vi "Main.vi"() -> ()   [LabVIEW 2020]
uses:
  States.ctl
  <vilib>/Instr/_visa.llb/VISA Configure Serial Port (Serial Instr).vi
  <vilib>/Utility/file.llb/Read Delimited Spreadsheet (I64).vi
panel:
  out "Next Control State":T1
  out "Next Com State":enum16{"Initialize", "Send", "Receive", "Error"}(ring)=enum."Receive"
  out "Next Cmd":enum16{"getParm", "inc", "mph", "err"}(ring)
  out "Send Buffer":string
  out "Control Error":errorcluster
  out "Com Error":errorcluster
  out "Missed Msg":u16
  out "Time Left":u32
  out "Inc Changed":bool
  out "Next MPH":u16
  out "Next Duration":u16
  out "Next Inc":u16
  out "PD READ":u8
  out "INC READ":u8
  out "MPH READ":u8
  out "dwell":u16[](array[numeric])
  out "incline":u16[](array[numeric])
  out "time":u16[](array[numeric])
  out "speed":u16[](array[numeric])
  out "input lines":i32
  in  "TestScript":path=path "C:/LabView Computer Backup SEAL2788/DonP_TRM500/FootTimeInc.txt"
  out "read buffer":string
  out "Speed Changed":bool
  in  "Manual Stop":bool
  in  "Serial Port":refnum<visa-resource-name>="COM8"
  out "FootPath":path
  out "FootPathRef":refnum<file>
  out "stopping":bool
  out "Target MPH":u16 max=12 step=1
  out "step":i32
  out "Target INC":u16 max=12 step=1
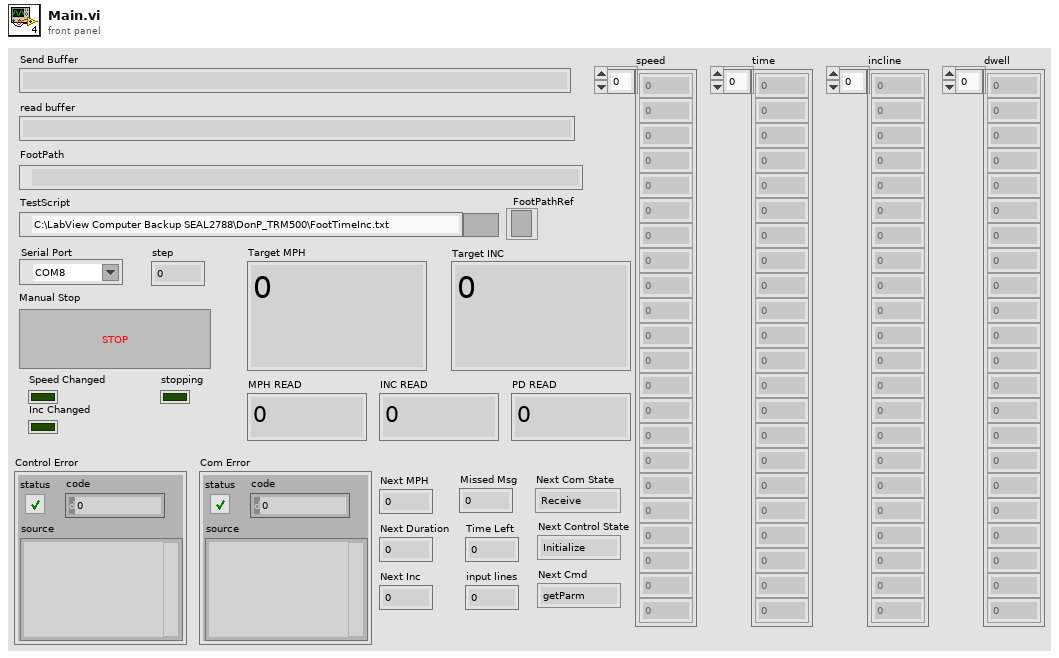
[diagram p1: front panel]
types:
  T1 = typedef "States.ctl" = enum16{"Initialize", "SetTargets", "WaitforMPH", "Dwell", "CheckTiming"}
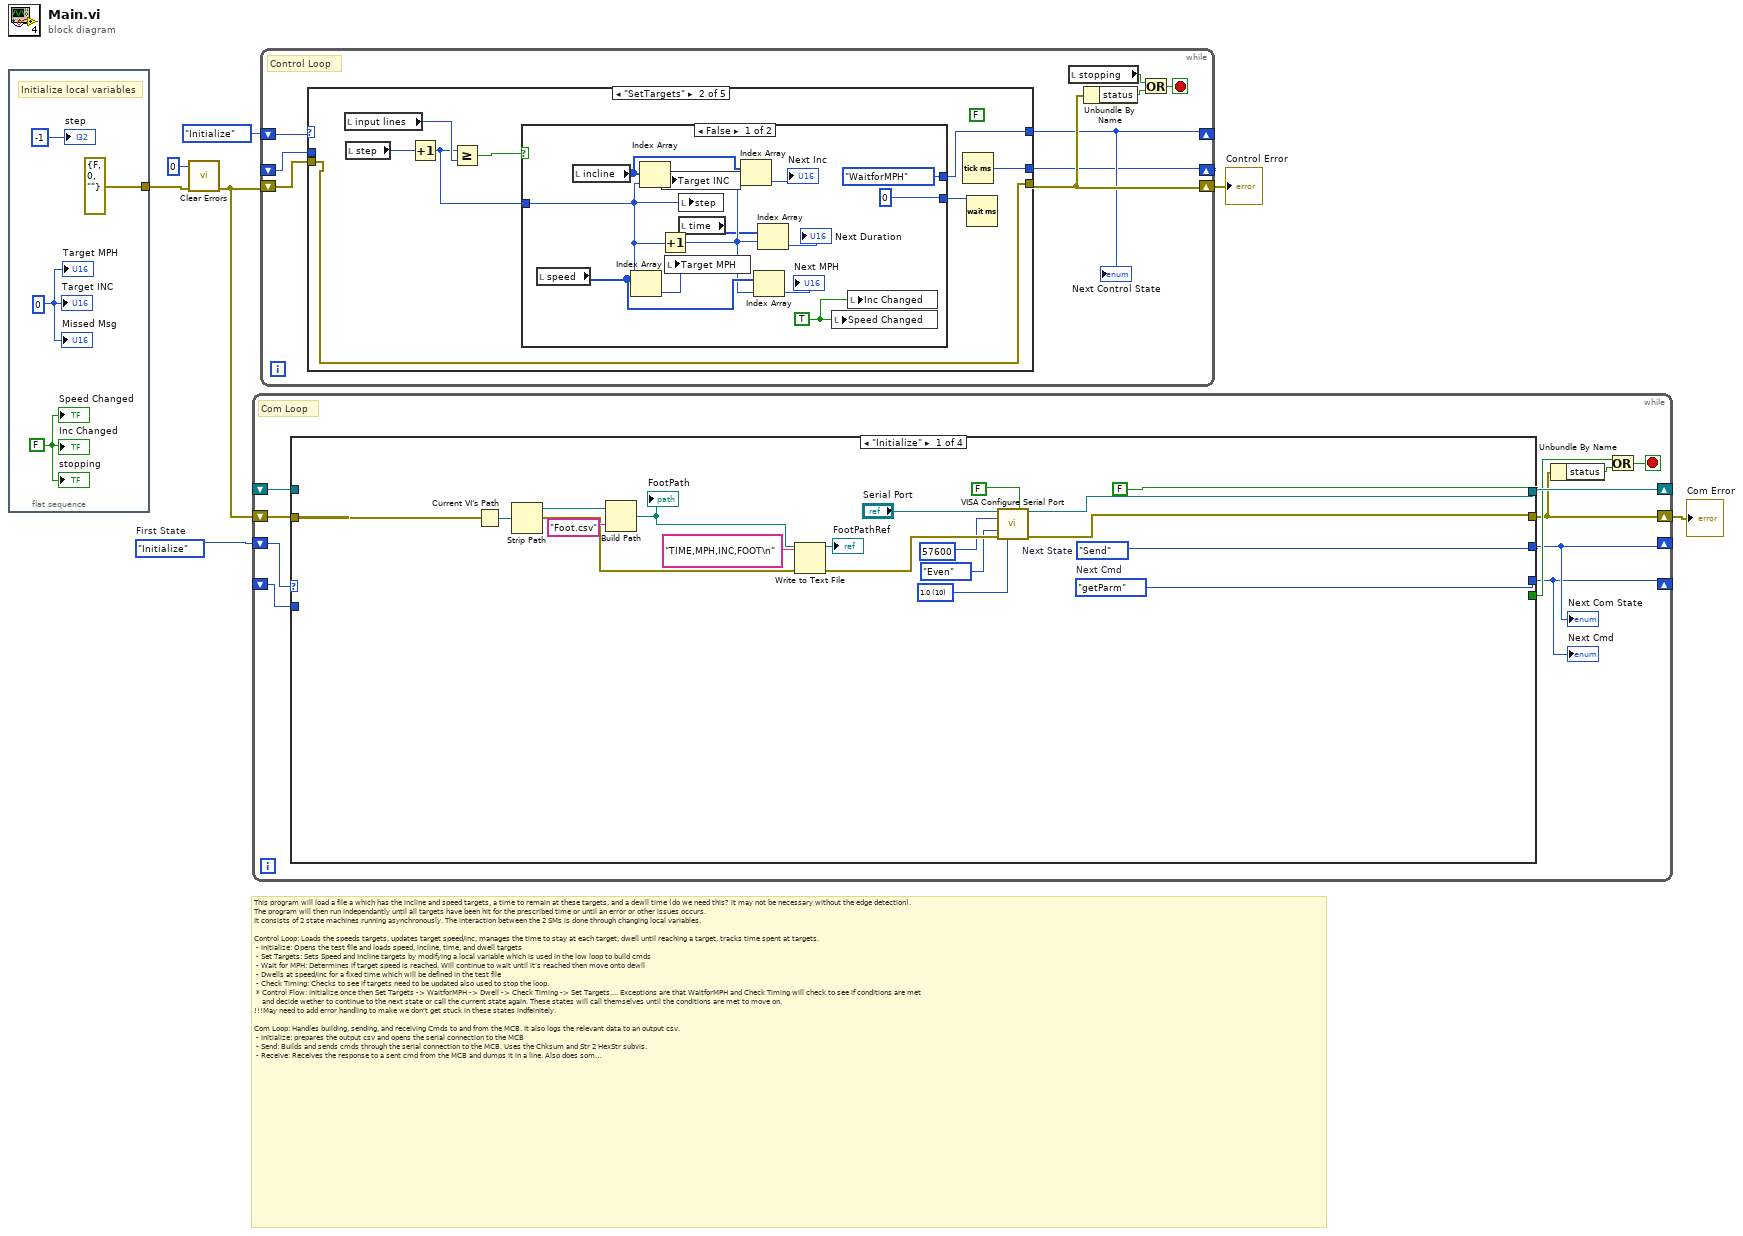
[diagram p0: block diagram]
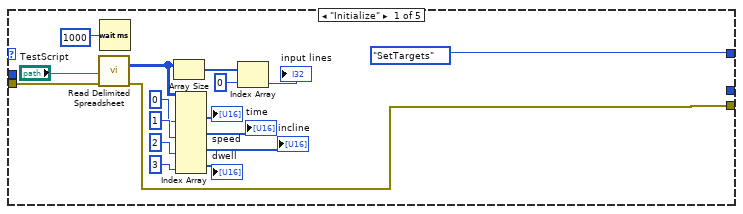
[diagram p2: hidden frame]
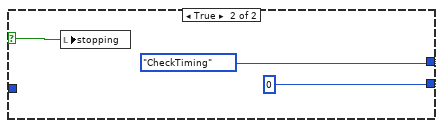
[diagram p3: hidden frame]
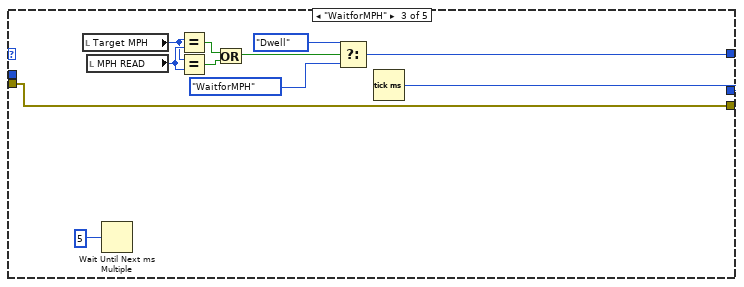
[diagram p4: hidden frame]
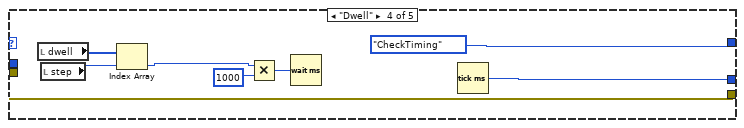
[diagram p5: hidden frame]
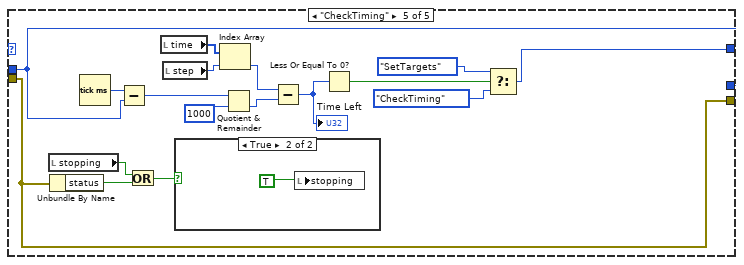
[diagram p6: hidden frame]
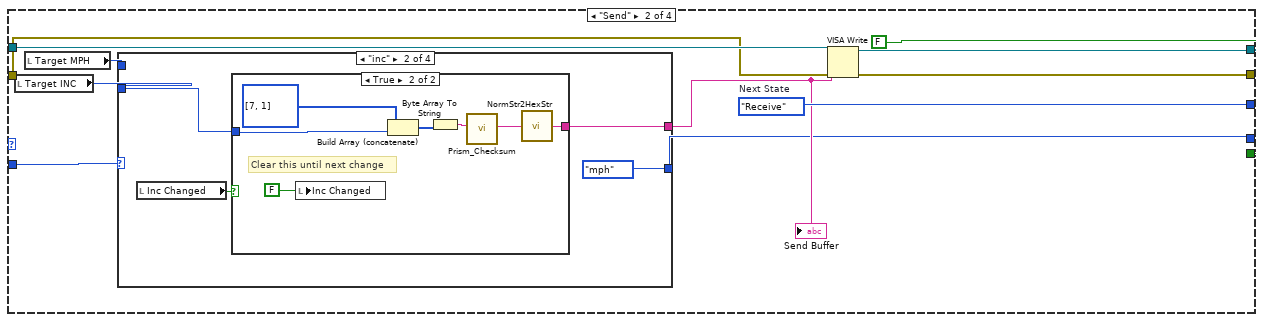
[diagram p8: hidden frame]
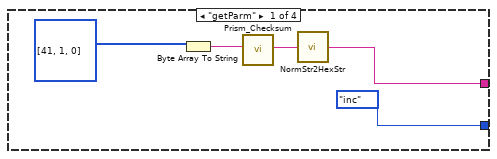
[diagram p9: hidden frame]
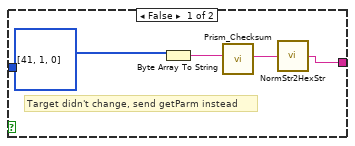
[diagram p10: hidden frame]
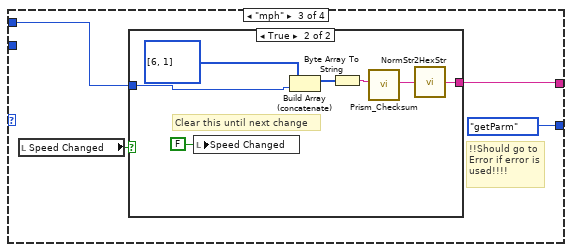
[diagram p11: hidden frame]
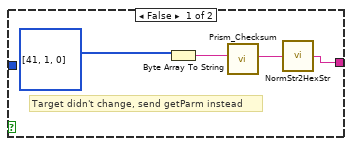
[diagram p12: hidden frame]
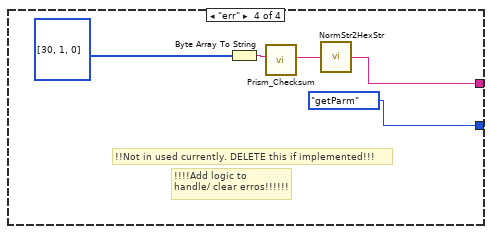
[diagram p13: hidden frame]
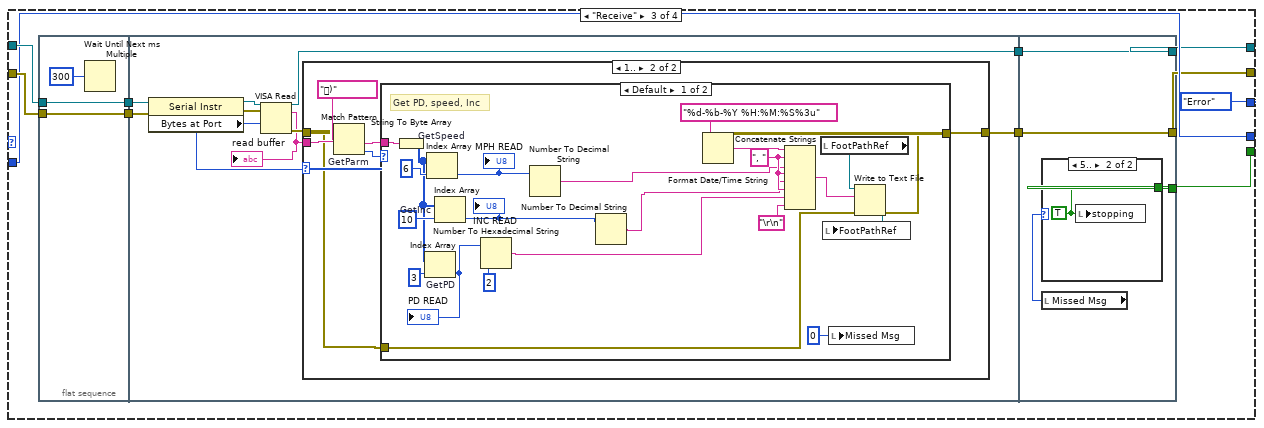
[diagram p14: hidden frame]
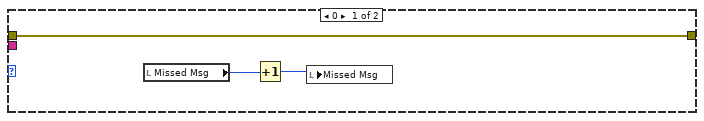
[diagram p15: hidden frame]
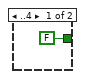
[diagram p17: hidden frame]
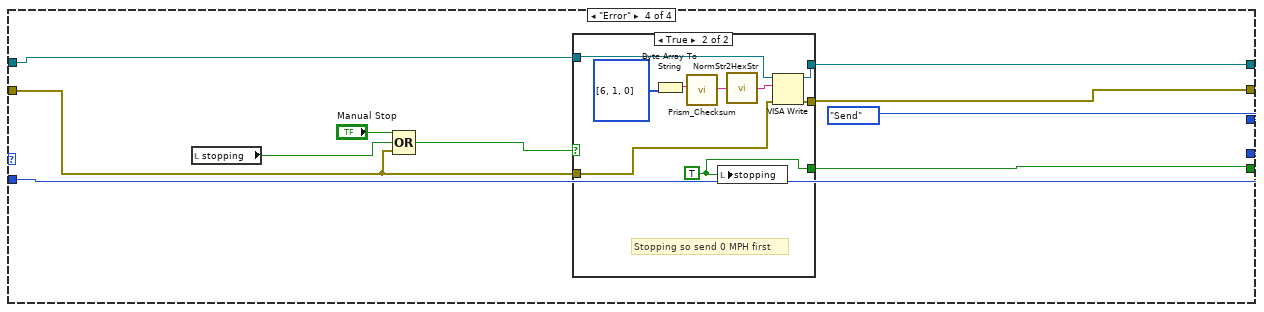
[diagram p18: hidden frame]
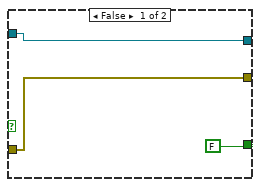
[diagram p19: hidden frame]
diagram:
  w7 = enum16{"Initialize", "Send", "Receive", "Error"}."Initialize"  # First State
  # "This program will load a file a which has the incline and speed targets, a time to remain at these targets, and a dewll time (do we need this? it may not be necessary without the edge detection).\nThe program will then run independantly until all targets have been hit for the prescribed time or until an error or other issues occurs.\nIt consists of 2 state machines running asynchronously. The interaction between the 2 SMs is done through changing local variables.\n\nControl Loop: Loads the speeds targets, updates target speed/inc, manages the time to stay at each target, dwell until reaching a target, tracks time spent at targets. \n - Initialize: Opens the test file and loads speed, incline, time, and dwell targets \n - Set Targets: Sets Speed and Incline targets by modifying a local variable which is used in the low loop to build cmds \n - Wait for MPH: Determines if target speed is reached. Will continue to wait until it's reached then move onto dewll\n - Dwells at speed/inc for a fixed time which will be defined in the test file\n - Check Timing: Checks to see if targets need to be updated also used to stop the loop.\n * Control Flow: Initialize once then Set Targets -> WaitforMPH -> Dwell -> Check Timing -> Set Targets.... Exceptions are that WaitforMPH and Check Timing will check to see if conditions are met\n    and decide wether to continue to the next state or call the current state again. These states will call themselves until the conditions are met to move on. \n!!!May need to add error handling to make we don't get stuck in these states indfeinitely.\n\nCom Loop: Handles building, sending, and receiving Cmds to and from the MCB. It also logs the relevant data to an output csv.\n - Initialize: prepares the output csv and opens the serial connection to the MCB\n - Send: Builds and sends cmds through the serial connection to the MCB. Uses the Chksum and Str 2 HexStr subvis. \n - Receive: Receives the response to a sent cmd from the MCB and dumps it in a line. Also does some analysis of the response to determine current  Speed/inc/person detect\n - Error:  Stops the program. This handles labview errors and will stop the program when one is encounted. It also handles stopping when reaching the end of a test \n * Com Flow: nitialize once then Send -> Receive -> Error -> Send...\n * Send flow: GetParm -> Inc -> MPH -> GetParm etc. Exception is that it will check first to see if the target changed and if it hasn't will send getParm Instead\n!!!May need to add error handling in which case the flow should be GetParm -> MPH -> Inc -> Err -> GetParm....\n\nFiles:\n1 input file which contains the test script to run. Format: Speed, Time, Inc, Dwell. Time = time to stay at target speed/inc. Dwell = a fixed time to wait after reaching targets and before starting the Time counter. This is used to make sure the speed stablizes before starting the Time counter.\n1 output file which contains Timestamp, Speed, Incline, and a flag for if person is detected (0 = No, 1 = Yes). Format: TIME,MPH,INC,FOOT"
  n1 = flat-sequence {
    tunnel: [errorcluster {"status"=FALSE, "code"=0, "source"=""} ("error constant")] -> w3
    frame #0 {
      w9 = FALSE ("Inc Changed")
      w8 = u16 0 ("MPH")
      # "Initialize local variables"
      "stopping" <- w9
      "Target MPH" <- w8
      "step" <- -1 ("step")
      "Target INC" <- w8
      "Speed Changed" <- w9
      "Inc Changed" <- w9
      "Missed Msg" <- w8
    }
  }
  n2 = call <vilib>:"Clear Errors.vi"("error in (no error)"=w3, "specific error code to clear (0: all)"=0) -> ("error out"=w2:errorcluster)  [unwired: 4 in, 1 out]
  n3 = while {
    shift-right: [w16] -> w6
    shift-left: w2 -> [w22]
    shift-right: [w19] -> _
    shift-left: _ -> [w21]
    shift-right: [w13] -> _
    shift-left: w7 -> [w20]
    shift-right: [w12] -> _
    shift-left: _ -> [w18]
    stop <- w15 stop-if-true
    # "Com Loop"
    n4 = case shown="\"Initialize\"" w20 {
      tunnel: w22 -> [w28 w42 w100 w156]
      tunnel: w21 -> [_ w49 w102 w154]
      tunnel: [w38 w51 w96 w153] -> w19
      tunnel: [w37 w50 w95 w155] -> w16
      tunnel: [w34 w45 enum16{"Initialize", "Send", "Receive", "Error"}."Error" enum16{"Initialize", "Send", "Receive", "Error"}."Send"] -> w13
      tunnel: [w36 w43 w99 w161] -> w12
      tunnel: w18 -> [_ w41 w99 w161]
      tunnel: [FALSE FALSE w92 w157] -> w17
      frame "Initialize" {
        w23 = u16 10 items=["1.0"=10, "1.5"=15, "2.0"=20] ("stop bits (10: 1 bit)")
        w34 = enum16{"Initialize", "Send", "Receive", "Error"}."Send"  # Next State
        w36 = enum16{"getParm", "inc", "mph", "err"}."getParm"  # Next Cmd
        n5 = Current VI's Path() -> (path=w33:path)
        n6 = Strip Path(path=w33) -> (stripped path=w32:path)  [unwired: 1 out]
        n7 = Build Path(base path=w32, name or relative path="Foot.csv") -> (appended path=w29:path)
        "FootPath" <- w29
        n8 = Write to Text File(file (use dialog)=w29, text="TIME,MPH,INC,FOOT\n", error in=w28) -> (refnum out=→"FootPathRef":refnum<file>, error out=w27:errorcluster)  [unwired: 1 in, 1 out]
        n9 = call-poly "VISA Configure Serial Port"("VISA resource name"="Serial Port", "Enable Termination\nChar (T)"=FALSE ("Enable Termination\nChar (T)"), "baud rate (9600)"=u32 57600, "parity (0:none)"=enum16{"None", "Odd", "Even", "Mark", "Space"}."Even", "error in (no error)"=w27, "stop bits (10: 1 bit)"=w23) -> ("VISA resource name out"=w38:refnum<visa-resource-name>, "error out"=w37:errorcluster)  [unwired: 8 in]
      }
      frame "Send" {
        w45 = enum16{"Initialize", "Send", "Receive", "Error"}."Receive"  # Next State
        n10 = local read "Target INC"() -> (w46:u16)
        n11 = local read "Target MPH"() -> (w47:u16)
        n12 = case shown="\"inc\"" w41 {
          tunnel: w47 -> [_ _ w73 _]
          tunnel: w46 -> [_ w60 _ _]
          tunnel: [w52 w59 w74 w88] -> w44
          tunnel: [enum16{"getParm", "inc", "mph", "err"}."inc" enum16{"getParm", "inc", "mph", "err"}."mph" enum16{"getParm", "inc", "mph", "err"}."getParm" enum16{"getParm", "inc", "mph", "err"}."getParm"] -> w43
          frame "getParm" {
            n13 = Byte Array To String(unsigned byte array=u8[] [41, 1, 0]) -> (string=w54:string)
            n14 = call "Prism_Checksum.vi"("ID +DB+ Data"=w54) -> ("Full Cmd"=w53:string)  [unwired: 10 in]
            n15 = call "NormStr2HexStr.vi"("string"=w53) -> ("hex string"=w52:string)
          }
          frame "inc" {
            n16 = local read "Inc Changed"() -> (w57:bool)
            n17 = case shown="True" w57 {
              tunnel: w60 -> [_ w68]
              tunnel: [w61 w66] -> w59
              frame False {
                # "Target didn't change, send getParm instead"
                n18 = Byte Array To String(unsigned byte array=u8[] [41, 1, 0]) -> (string=w63:string)
                n19 = call "Prism_Checksum.vi"("ID +DB+ Data"=w63) -> ("Full Cmd"=w62:string)  [unwired: 10 in]
                n20 = call "NormStr2HexStr.vi"("string"=w62) -> ("hex string"=w61:string)
              }
              frame True {
                # "Clear this until next change"
                n21 = local write "Inc Changed"(FALSE ("Value Changed")) -> ()
                n22 = Build Array (concatenate)(u8[] [7, 1] ("unsigned byte array"), w68) -> (w67:u16[])
                n23 = Byte Array To String(unsigned byte array=w67) -> (string=w70:string)
                n24 = call "Prism_Checksum.vi"("ID +DB+ Data"=w70) -> ("Full Cmd"=w71:string)  [unwired: 10 in]
                n25 = call "NormStr2HexStr.vi"("string"=w71) -> ("hex string"=w66:string)
              }
            }
          }
          frame "mph" {
            # "!!Should go to\nError if error is\nused!!!!"
            n26 = local read "Speed Changed"() -> (w72:bool)
            n27 = case shown="True" w72 {
              tunnel: [w76 w83] -> w74
              tunnel: w73 -> [_ w81]
              frame False {
                # "Target didn't change, send getParm instead"
                n28 = Byte Array To String(unsigned byte array=u8[] [41, 1, 0]) -> (string=w78:string)
                n29 = call "Prism_Checksum.vi"("ID +DB+ Data"=w78) -> ("Full Cmd"=w77:string)  [unwired: 10 in]
                n30 = call "NormStr2HexStr.vi"("string"=w77) -> ("hex string"=w76:string)
              }
              frame True {
                # "Clear this until next change"
                n31 = local write "Speed Changed"(FALSE ("Value Changed")) -> ()
                n32 = Build Array (concatenate)(u8[] [6, 1] ("unsigned byte array"), w81) -> (w82:u16[])
                n33 = Byte Array To String(unsigned byte array=w82) -> (string=w85:string)
                n34 = call "Prism_Checksum.vi"("ID +DB+ Data"=w85) -> ("Full Cmd"=w86:string)  [unwired: 10 in]
                n35 = call "NormStr2HexStr.vi"("string"=w86) -> ("hex string"=w83:string)
              }
            }
          }
          frame "err" {
            # "!!Not in used currently. DELETE this if implemented!!!"
            # "!!!!Add logic to\nhandle/ clear erros!!!!!!"
            n36 = Byte Array To String(unsigned byte array=u8[] [30, 1, 0]) -> (string=w90:string)
            n37 = call "Prism_Checksum.vi"("ID +DB+ Data"=w90) -> ("Full Cmd"=w91:string)  [unwired: 10 in]
            n38 = call "NormStr2HexStr.vi"("string"=w91) -> ("hex string"=w88:string)
          }
        }
        "Send Buffer" <- w44
        n39 = VISA Write(VISA resource name=w49, write buffer=w44, error in (no error)=w42) -> (VISA resource name out=w51:refnum<visa-resource-name>, error out=w50:errorcluster)  [unwired: 1 out]
      }
      frame "Receive" {
        n40 = flat-sequence {
          tunnel: w102 -> [w104]
          tunnel: w100 -> [w103]
          tunnel: [w104] -> w98
          tunnel: [w103] -> w97
          tunnel: w98 -> [w114]
          tunnel: w97 -> [w113]
          tunnel: [w106] -> w94
          tunnel: [w110] -> w93
          tunnel: [w149] -> w95
          tunnel: [w150] -> w96
          tunnel: w94 -> [w150]
          tunnel: w93 -> [w149]
          tunnel: [w147] -> w92
          frame #0 {
            n41 = Wait Until Next ms Multiple(millisecond multiple=u32 300) -> ()  [unwired: 1 out]
          }
          frame #1 {
            n42 = property class="Serial Instr"(reference=w114, error in=w113) -> (reference out=w111:refnum<visa-resource-name>, error out=w112:errorcluster, "Bytes at Port"=w109:u32)
            n43 = VISA Read(VISA resource name=w111, byte count=w109, error in (no error)=w112) -> (VISA resource name out=w106:refnum<visa-resource-name>, read buffer=w107:string, error out=w108:errorcluster)  [unwired: 1 out]
            "read buffer" <- w107
            n44 = case shown="1.." w109 {
              tunnel: [w117 w119] -> w110
              tunnel: w108 -> [w117 w118]
              tunnel: w107 -> [_ w120]
              frame 0 {
                n45 = local read "Missed Msg"() -> (w116:u16)
                n46 = Increment(x=w116) -> (x+1=w115:u16)
                n47 = local write "Missed Msg"(w115) -> ()
              }
              frame 1.. {
                n48 = Match Pattern "GetParm"(string=w120, regular expression="ޭ)") -> (after substring=w122:string, offset past match=w121:i32)  [unwired: 1 in, 2 out]
                n49 = case shown="Default" w121 {
                  tunnel: w122 -> [w141 _]
                  tunnel: [w138 w146] -> w119
                  tunnel: w118 -> [w133 w146]
                  frame Default {
                    w131 = ", "
                    # "Get PD, speed, Inc"
                    n50 = String To Byte Array(string=w141) -> (unsigned byte array=w142:u8[])
                    n51 = Index Array "GetPD"(array=w142, index=3) -> (element=w135:u8)
                    "PD READ" <- w135
                    n52 = Index Array "GetSpeed"(array=w142, index=6) -> (element=w125:u8)
                    "MPH READ" <- w125
                    n53 = Index Array "GetInc"(array=w142, index=10) -> (element=w124:u8)
                    "INC READ" <- w124
                    n54 = Number To Hexadecimal String(1:i16 2 ("width (-)"), 2:w135) -> (0:w128:string)
                    n55 = Number To Decimal String(number=w125) -> (decimal integer string=w127:string)  [unwired: 1 in]
                    n56 = Number To Decimal String(number=w124) -> (decimal integer string=w126:string)  [unwired: 1 in]
                    n57 = Format Date/Time String(time format string (%c)="%d-%b-%Y %H:%M:%S%3u") -> (date/time string=w136:string)  [unwired: 2 in]
                    n58 = Concatenate Strings(w136, w131, w127, w131, w126, w131, w128, "\r\n") -> (w139:string)
                    n59 = local read "FootPathRef"() -> (w137:refnum<file>)
                    n60 = local write "Missed Msg"(u16 0 ("Missed Msg")) -> ()
                    n61 = Write to Text File(file (use dialog)=w137, text=w139, error in=w133) -> (refnum out=w129:refnum<file>, error out=w138:errorcluster)  [unwired: 1 in, 1 out]
                    n62 = local write "FootPathRef"(w129) -> ()
                  }
                  frame -1 {
                  }
                }
              }
            }
          }
          frame #2 {
            n63 = local read "Missed Msg"() -> (w148:u16)
            n64 = case shown="5.." w148 {
              tunnel: [FALSE ("stopping") w152] -> w147
              frame ..4 {
              }
              frame 5.. {
                w152 = TRUE ("stopping")
                n65 = local write "stopping"(w152) -> ()
              }
            }
          }
        }
      }
      frame "Error" {
        n66 = local read "stopping"() -> (w158:bool)
        n67 = Compound Arithmetic op=OR("Manual Stop", w158, w156) -> (w160:bool)
        n68 = case shown="True" w160 {
          tunnel: [FALSE w174] -> w157
          tunnel: w156 -> [w164 w169]
          tunnel: [w164 w168] -> w155
          tunnel: w154 -> [w163 w167]
          tunnel: [w163 w166] -> w153
          frame False {
          }
          frame True {
            w174 = TRUE ("stopping")
            # "Stopping so send 0 MPH first"
            n69 = Byte Array To String(unsigned byte array=u8[] [6, 1, 0]) -> (string=w173:string)
            n70 = call "Prism_Checksum.vi"("ID +DB+ Data"=w173) -> ("Full Cmd"=w172:string)  [unwired: 10 in]
            n71 = local write "stopping"(w174) -> ()
            n72 = call "NormStr2HexStr.vi"("string"=w172) -> ("hex string"=w171:string)
            n73 = VISA Write(VISA resource name=w167, write buffer=w171, error in (no error)=w169) -> (VISA resource name out=w166:refnum<visa-resource-name>, error out=w168:errorcluster)  [unwired: 1 out]
          }
        }
      }
    }
    "Next Com State" <- w13
    "Next Cmd" <- w12
    n74 = Unbundle By Name(w16) -> ("status"=w14:bool)
    n75 = Or(x=w17, y=w14) -> (x .or. y?=w15:bool)
  }
  "Com Error" <- w6
  n76 = while {
    shift-right: [w180] -> w5
    shift-left: w2 -> [w183]
    shift-right: [w178] -> _
    shift-left: _ -> [w177]
    shift-right: [w179] -> _
    shift-left: States."Initialize" ("First State") -> [w176]
    stop <- w181 stop-if-true
    # "Control Loop"
    n77 = case shown="\"SetTargets\"" w176 {
      tunnel: w183 -> [w198 w201 w234 w240 w244]
      tunnel: [w188 w201 w234 w240 w244] -> w180
      tunnel: [States."SetTargets" ("First State") w205 w232 States."CheckTiming" ("First State") w245] -> w179
      tunnel: [_ w203 w233 w237 w256] -> w178
      tunnel: w177 -> [_ _ _ _ w256]
      frame "Initialize" {
        n78 = call-poly <vilib>:"Read Delimited Spreadsheet.vi"("file path (dialog if empty)"="TestScript", "error in (no error)"=w198) -> ("all rows"=w194:i64[][], "error out"=w188:errorcluster)  [unwired: 8 in, 4 out]
        n79 = Wait (ms)(milliseconds to wait=u32 1000) -> ()  [unwired: 1 out]
        n80 = Array Size(array=w194) -> (size(s)=w196:i32[])
        n81 = Index Array(array=w194, index (col) #1=0 ("index"), index (col) #2=1 ("index (col)"), index (col) #3=2 ("index (col)"), index (col) #4=3 ("index (col)")) -> (element #1=→"speed":i64[], element #2=→"time":i64[], element #3=→"incline":i64[], element #4=→"dwell":i64[])  [unwired: 4 in]
        n82 = Index Array(array=w196, index=0) -> (element=→"input lines":i32)
      }
      frame "SetTargets" {
        (unwired) FALSE
        n83 = local read "input lines"() -> (w207:i32)
        n84 = local read "step"() -> (w208:i32)
        n85 = Increment(x=w208) -> (x+1=w202:i32)
        n86 = Greater Or Equal?(x=w202, y=w207) -> (x >= y?=w206:bool)
        n87 = case shown="False" w206 {
          selector: w206 -> [_ w224]
          tunnel: [States."WaitforMPH" ("First State") States."CheckTiming" ("First State")] -> w205
          tunnel: [u32 0 ("milliseconds to wait") u32 0 ("milliseconds to wait")] -> w204
          tunnel: w202 -> [w219 _]
          frame False {
            w210 = TRUE ("Value Changed")
            n88 = local read "speed"() -> (w218:u16[])
            n89 = local read "incline"() -> (w217:u16[])
            n90 = Index Array(array=w218, index=w219) -> (element=w221:u16)
            n91 = Index Array(array=w217, index=w219) -> (element=w220:u16)
            n92 = Increment(x=w219) -> (x+1=w216:i32)
            n93 = local write "Target INC"(w220) -> ()
            n94 = local write "Target MPH"(w221) -> ()
            n95 = local write "step"(w219) -> ()
            n96 = local read "time"() -> (w215:u16[])
            n97 = Index Array(array=w217, index=w216) -> (element=→"Next Inc":u16)
            n98 = Index Array(array=w218, index=w216) -> (element=→"Next MPH":u16)
            n99 = Index Array(array=w215, index=w216) -> (element=→"Next Duration":u16)
            n100 = local write "Speed Changed"(w210) -> ()
            n101 = local write "Inc Changed"(w210) -> ()
          }
          frame True {
            n102 = local write "stopping"(w224) -> ()
          }
        }
        n103 = Tick Count (ms)() -> (millisecond timer value=w203:u32)
        n104 = Wait (ms)(milliseconds to wait=w204) -> ()  [unwired: 1 out]
      }
      frame "WaitforMPH" {
        n105 = local read "Target MPH"() -> (w227:u16)
        n106 = local read "MPH READ"() -> (w228:u8)
        n107 = Wait Until Next ms Multiple(millisecond multiple=u32 5) -> ()  [unwired: 1 out]
        n108 = Equal?(x=w227, y=w228) -> (x = y?=w230:bool)
        n109 = Equal?(x=w227, y=w228) -> (x = y?=w229:bool)
        n110 = Or(x=w230, y=w229) -> (x .or. y?=w231:bool)
        n111 = Select(t=States."Dwell" ("First State"), s=w231, f=States."WaitforMPH" ("First State")) -> (s? t:f=w232:T1)
        n112 = Tick Count (ms)() -> (millisecond timer value=w233:u32)
      }
      frame "Dwell" {
        n113 = local read "dwell"() -> (w238:u16[])
        n114 = local read "step"() -> (w239:i32)
        n115 = Index Array(array=w238, index=w239) -> (element=w243:u16)
        n116 = Multiply(x=w243, y=u16 1000) -> (x*y=w241:u16)
        n117 = Wait (ms)(milliseconds to wait=w241) -> ()  [unwired: 1 out]
        n118 = Tick Count (ms)() -> (millisecond timer value=w237:u32)
      }
      frame "CheckTiming" {
        n119 = local read "stopping"() -> (w258:bool)
        n120 = Unbundle By Name(w244) -> ("status"=w259:bool)
        n121 = Tick Count (ms)() -> (millisecond timer value=w260:u32)
        n122 = Subtract(x=w260, y=w256) -> (x-y=w255:u32)
        n123 = Or(x=w258, y=w259) -> (x .or. y?=w257:bool)
        n124 = local read "time"() -> (w253:u16[])
        n125 = local read "step"() -> (w252:i32)
        n126 = case shown="True" w257 {
          frame False {
          }
          frame True {
            n127 = local write "stopping"(TRUE ("stopping")) -> ()
          }
        }
        n128 = Index Array(array=w253, index=w252) -> (element=w250:u16)
        n129 = Quotient & Remainder(x=w255, y=u32 1000) -> (floor(x/y)=w251:u32)  [unwired: 1 out]
        n130 = Subtract(x=w250, y=w251) -> (x-y=w249:u32)
        "Time Left" <- w249
        n131 = Less Or Equal To 0?(x=w249) -> (x <= 0?=w248:bool)
        n132 = Select(t=States."SetTargets" ("First State"), s=w248, f=States."CheckTiming" ("First State")) -> (s? t:f=w245:T1)
      }
    }
    "Next Control State" <- w179
    n133 = local read "stopping"() -> (w175:bool)
    n134 = Unbundle By Name(w180) -> ("status"=w182:bool)
    n135 = Or(x=w175, y=w182) -> (x .or. y?=w181:bool)
  }
  "Control Error" <- w5
